vi "BackToPanel.vi"(8 "error in (no error)":errorcluster caption="错误输入（无错误）", 11 "PanelDataNode 输入":refnum<class "PanelDataNode.lvclass"> caption="DNL_LabVIEW Object in") -> (0 "error out":errorcluster caption="错误输出", 3 "PanelDataNode 输出":refnum<class "PanelDataNode.lvclass"> caption="DNL_LabVIEW Object out")   [LabVIEW 2013, in "PanelDataNode.lvclass"]
uses:
  PanelDataNode.lvclass
  PanelDataNode.lvclass/PanelDataNode.ctl
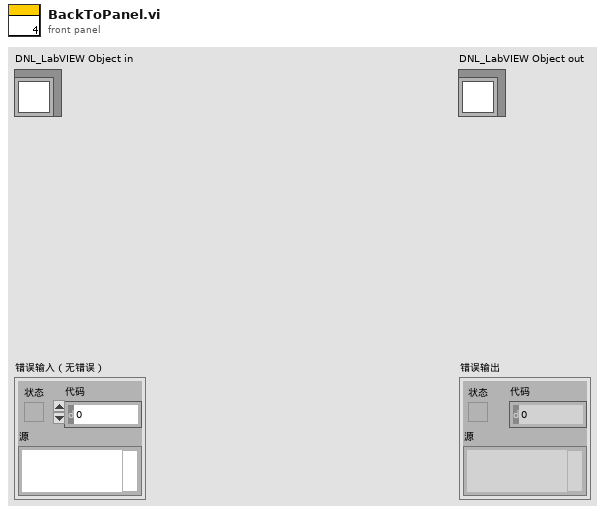
[diagram p1: front panel]
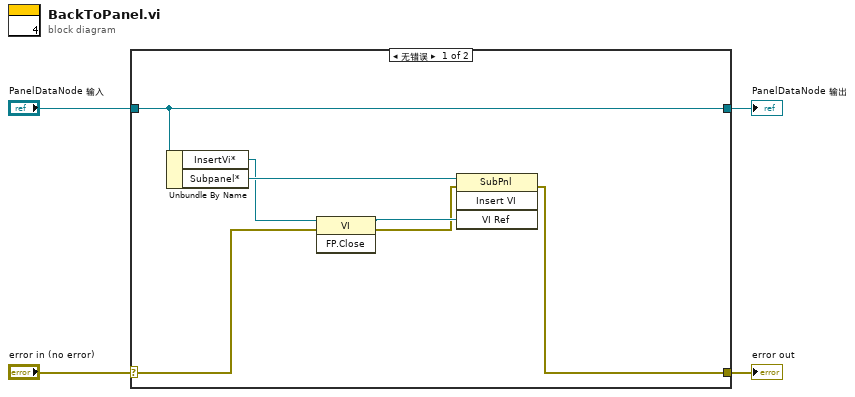
[diagram p0: block diagram]
diagram:
  n1 = case shown="无错误" "error in (no error)" {
    selector: "error in (no error)" -> [w6 w13]
    tunnel: [w9 w13] -> w3
    tunnel: [w11 w12] -> w1
    tunnel: "PanelDataNode 输入" -> [w11 w12]
    frame No Error {
      n2 = Unbundle By Name(w11) -> ("InsertVi*"=w8:refnum<vi>, "Subpanel*"=w10:refnum<vi>)
      n3 = invoke class="VI" method="FP.Close"(reference=w8, error in=w6) -> (reference out=w7:refnum<vi>, error out=w5:errorcluster)  [unwired: 1 in, 1 out]
      n4 = invoke class="SubPnl" method="Insert VI"(reference=w10, error in=w5, "VI Ref"=w7) -> (error out=w9:errorcluster)  [unwired: 1 in, 3 out]
    }
    frame Error {
    }
  }
  "error out" <- w3
  "PanelDataNode 输出" <- w1
